vi "220401_Basic1.vi"() -> ()   [LabVIEW 2021]
panel:
  in  "Textwarning":string
  out "?":bool
  out "?":bool
  out "Numeric":u64
  in  "stop":bool
  out "Tank":dbl(slide) scale=0.0..1000.0
  in  "Wert2":i8(knob) scale=0.0..10.0
  in  "Wert1":dbl(knob) scale=0.0..100.0
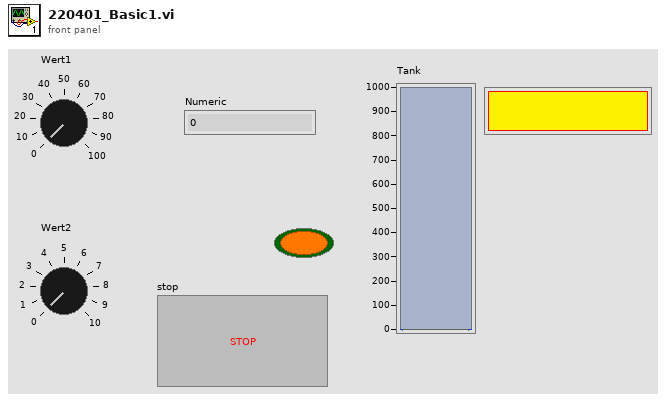
[diagram p1: front panel]
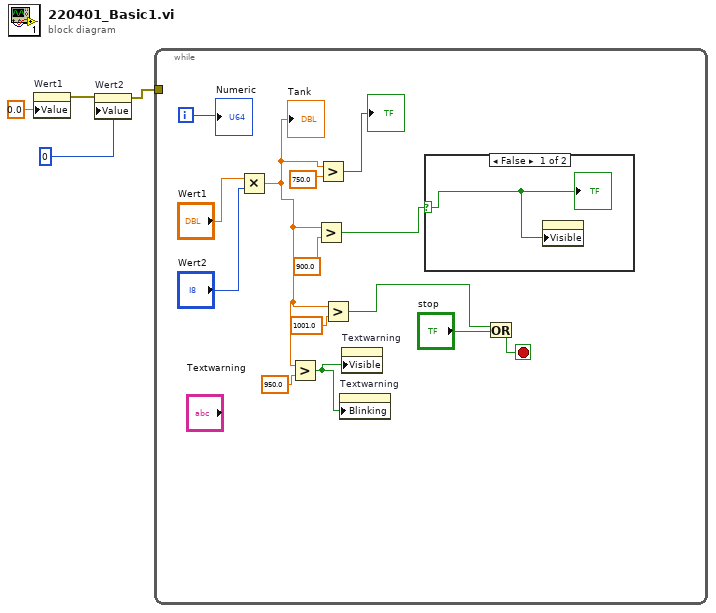
[diagram p0: block diagram]
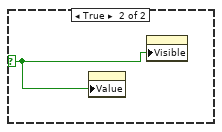
[diagram p2: hidden frame]
diagram:
  n1 = property on="Wert1" class="Knob (strict)"("Value"=0.0 ("Wert1")) -> (error out=w2:errorcluster)  [unwired: 2 in, 1 out]
  n2 = property on="Wert2" class="Knob (strict)"(error in=w2, "Value"=i8 0 ("Wert2")) -> (error out=w1:errorcluster)  [unwired: 1 in, 1 out]
  n3 = while {
    tunnel: w1 -> [_]
    i -> [w18]
    stop <- w12 stop-if-true
    n4 = Multiply(x="Wert1", y="Wert2") -> (x*y=w7:dbl)
    "Tank" <- w7
    n5 = Greater?(x=w7, y=950.0) -> (0:w6:bool)
    n6 = Greater?(x=w7, y=900.0) -> (0:w8:bool)
    n7 = Greater?(x=w7, y=750.0) -> (0:→"?":bool)
    n8 = Greater?(x=w7, y=1001.0) -> (0:w10:bool)
    n9 = property on="Textwarning" class="Str"("Blinking"=w6) -> ()  [unwired: 2 in, 2 out]
    n10 = property on="Textwarning" class="Str"("Visible"=w6) -> ()  [unwired: 2 in, 2 out]
    n11 = case shown="False" w8 {
      selector: w8 -> [w19 w20]
      frame False {
        n12 = property class="Bool (strict)"("Visible"=w19) -> ()  [unwired: 2 in, 2 out]
        "?" <- w19
      }
      frame True {
        n13 = property class="Bool (strict)"("Value"=w20) -> ()  [unwired: 2 in, 2 out]
        n14 = property class="Bool (strict)"("Visible"=w20) -> ()  [unwired: 2 in, 2 out]
      }
    }
    n15 = Or(x=w10, y="stop") -> (x .or. y?=w12:bool)
    "Numeric" <- w18
  }
